vi "DataPacker_ReadMIDASAddress.vi"(8 "error in (no error)":errorcluster, 11 "DataPacker in":refnum<class "DataPacker.lvclass">) -> (0 "error out":errorcluster, 2 "Address to Log To":u32, 3 "DataPacker out":refnum<class "DataPacker.lvclass">)   [LabVIEW 2018, in "feGEM DataPacker.lvlib" / "DataPacker.lvclass"]
uses:
  DataPacker.lvclass
  DataPacker.lvclass/DataPacker.ctl
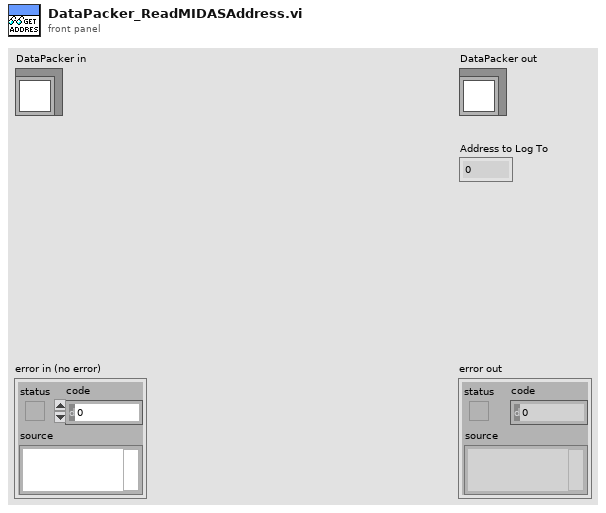
[diagram p1: front panel]
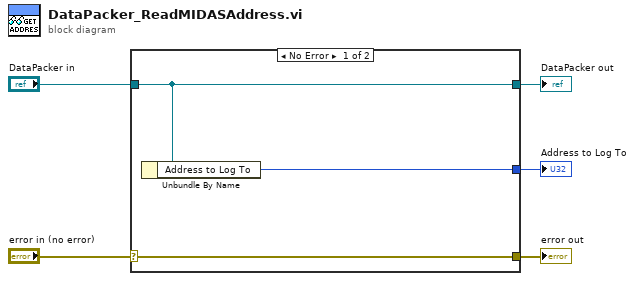
[diagram p0: block diagram]
diagram:
  n1 = case shown="No Error" "error in (no error)" {
    selector: "error in (no error)" -> [w8 w9]
    tunnel: [w8 w9] -> w4
    tunnel: [w7 w10] -> w2
    tunnel: "DataPacker in" -> [w7 w10]
    tunnel: [w6 _] -> w1
    frame No Error {
      n2 = Unbundle By Name(w7) -> ("Address to Log To"=w6:u32)
    }
    frame Error {
    }
  }
  "error out" <- w4
  "DataPacker out" <- w2
  "Address to Log To" <- w1
